vi "Sequence Execution.vi"() -> ()   [LabVIEW 2013, in "Simple Sequence Tools - Execution.lvlib"]
uses:
  Simple Sequence Tools - Execution.lvlib
  Types/Log.SelectedChannels.ctl
  Types/Execute.PreviewMode.ctl
  Types/Main.StateVariables.ctl
  Types/Execute.UserEventRefs.ctl
  <vilib>/NI Veristand/Execution/Workspace/SystemStateRegEventRef.ctl
  Types/Execution.SequenceState.ctl
  <vilib>/NI Veristand/Execution/DataLogging/DataLoggingSpecification Ref.ctl
  <vilib>/NI Veristand/Execution/DataLogging/IDataLogging Ref.ctl
  <vilib>/NI Veristand/Execution/Workspace/WorkspaceAPI.ctl
  <vilib>/NI Veristand/Execution/Workspace/SystemStateEventRef.ctl
  Shared/Types/INI.Settings
  NationalInstruments.VeriStand.RealTimeSequenceDefinitionApi
  Types/Results.Value.ctl
  Shared/SubVIs/Main.Constants.vi
  <vilib>/NI Veristand/Execution/Workspace/NI VeriStand - Set Single Channel Value.vi
  <vilib>/NI Veristand/Execution/Workspace/NI_VS Workspace ExecutionAPI.lvlib
  NationalInstruments.VeriStand.ClientAPI
  Shared/Simple Sequence Tools - Shared.lvlib
  <vilib>/NI Veristand/Execution/DataLogging/NI_VS Data Logging API.lvlib
panel:
  out "Duration":dbl min=1.0 max=3.0
  in  "Skip":bool
  out "Total Iterations":u32 min=1 max=2
  out "Current Step":u32 min=1 max=5
  out "Current Iteration":u32 min=1 max=2
  in  "NIVS.Gateway IP Address":string="localhost"
  in  "NIVS.Workspace Event":refnum<event-registration>
  in  "Preview Mode":T1=enum."Table"
  in  "Start Step":u32 min=1 max=11
  in  "Start Iteration":u32 min=1 max=5
  in  "Log Channels":T2=enum."Aliases"
  in  "Base File Name":string="Log" caption="Base File Name (timestamp included automatically)"
  in  "Enable Logging":bool=TRUE
  in  "Abort":bool
  in  "Pause":bool
  in  "Run":bool
  in  "Profiles":string(combo)
  out "Graph":waveform(dbl)[](graph)
  out "Sequence":i32[](listbox)=[-1]
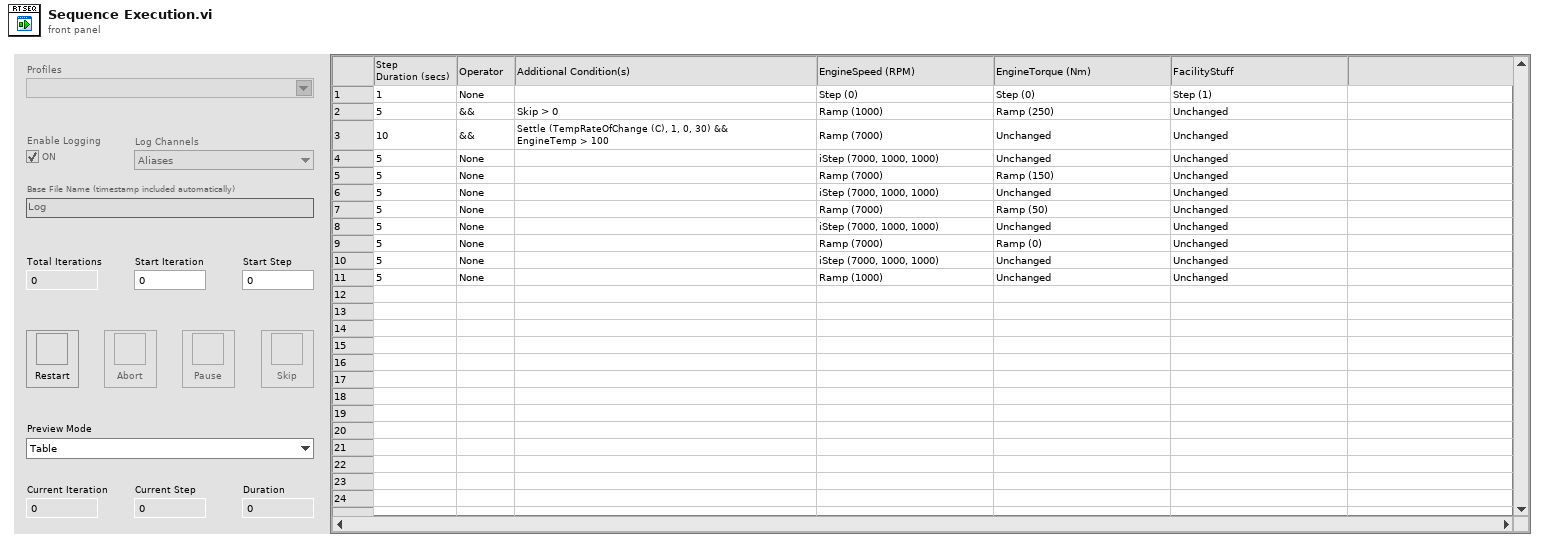
[diagram p1: front panel]
types:
  T1 = typedef "Simple Sequence Tools - Execution.lvlib/Execute.PreviewMode.ctl" = enum8{"Graph", "Table"}
  T2 = typedef "Simple Sequence Tools - Execution.lvlib/Log.SelectedChannels.ctl" = enum16{"Channels (No System Channel)", "Aliases", "All"}
  T3 = typedef "Simple Sequence Tools - Execution.lvlib/Execution.SequenceState.ctl" = enum16{"Idle", "Initializing", "Running", "Paused", "Finalizing", "Complete"}
  T4 = typedef "Simple Sequence Tools - Execution.lvlib/Main.StateVariables.ctl" = cluster{"NIVS.BaseLogPath":path, "NIVS.SystemDefinitionFile":path, "NIVS.Events":T5, "NIVS.SequenceState":T3, "NIVS.GatewayIPAddress":string, "NIVS.DataLogSpecRef":T7, "NIVS.DataLogManagerRef":T8, "NIVS.LogSessionGUID":string, "NIVS.WorkspaceManager":T9, "NIVS.Deployed":bool, "NIVS.ProfileRef":refnum<k24>, "NIVS.ProfileCallback":refnum<k27>, "NIVS.SystemStateRefs":T10, "UI.Abort":refnum<vi>, "UI.Pause":refnum<vi>, "UI.EnableLogging":refnum<vi>, "UI.Start":refnum<vi>, "UI.LogChannels":refnum<vi>, "UI.StartIteration":refnum<vi>, "UI.StartStep":refnum<vi>, "UI.Sequence":refnum<vi>, "UI.PreviewMode":refnum<vi>, "UI.Graph":refnum<vi>, "UI.BaseFileName":refnum<vi>, "UI.Profiles":refnum<vi>, "UI.CurrentStep":refnum<vi>, "UI.CurrentIteration":refnum<vi>, "UI.TotalIterations":refnum<vi>, "Sequence.AbortChannel":string, "Sequence.StepInfoChannel":string, "Sequence.Iterations":u32, "Sequence.IterationInfoChannel":string, "Sequence.#ofColumns":i32, "Events.State":refnum<user-event>, "Events.Test Result":refnum<user-event>, "Events.Progress":refnum<user-event>, "INI.Settings":T11, "UI.Skip":refnum<vi>, "Sequence.SkipChannel":string, "Restart.Path":path, "UI.Duration":refnum<vi>, "Sequence.DurationChannel":string}
  T5 = typedef "Simple Sequence Tools - Execution.lvlib/Execute.UserEventRefs.ctl" = cluster{"SequenceEvent":refnum<event-registration>, "SystemChangeEvent":T6, "WorkspaceEvent":refnum<event-registration>}
  T6 = typedef "NI_VS Workspace ExecutionAPI.lvlib/SystemStateRegEventRef.ctl" = refnum<event-registration>
  T7 = typedef "NI_VS Data Logging API.lvlib/DataLoggingSpecification Ref.ctl" = refnum<k24>
  T8 = typedef "NI_VS Data Logging API.lvlib/IDataLogging Ref.ctl" = refnum<k24>
  T9 = typedef "NI_VS Workspace ExecutionAPI.lvlib/WorkspaceAPI.ctl" = refnum<k24>
  T10 = typedef "NI_VS Workspace ExecutionAPI.lvlib/SystemStateEventRef.ctl" = cluster{"CustDatRef":refnum<user-event>, "EvtRef":refnum<k27>}
  T11 = typedef "Simple Sequence Tools - Shared.lvlib/INI.Settings" = cluster{"Build Location":path, "LoggingLocation":path}
  T12 = typedef "Simple Sequence Tools - Execution.lvlib/Results.Value.ctl" = enum8{"Passed", "Failed", "Aborted"}
  T13 = enum8{"Enabled", "Disabled", "Disabled and Grayed Out"}
  T14 = typedef "NI_VS Workspace ExecutionAPI.lvlib/SystemState.ctl" = u8
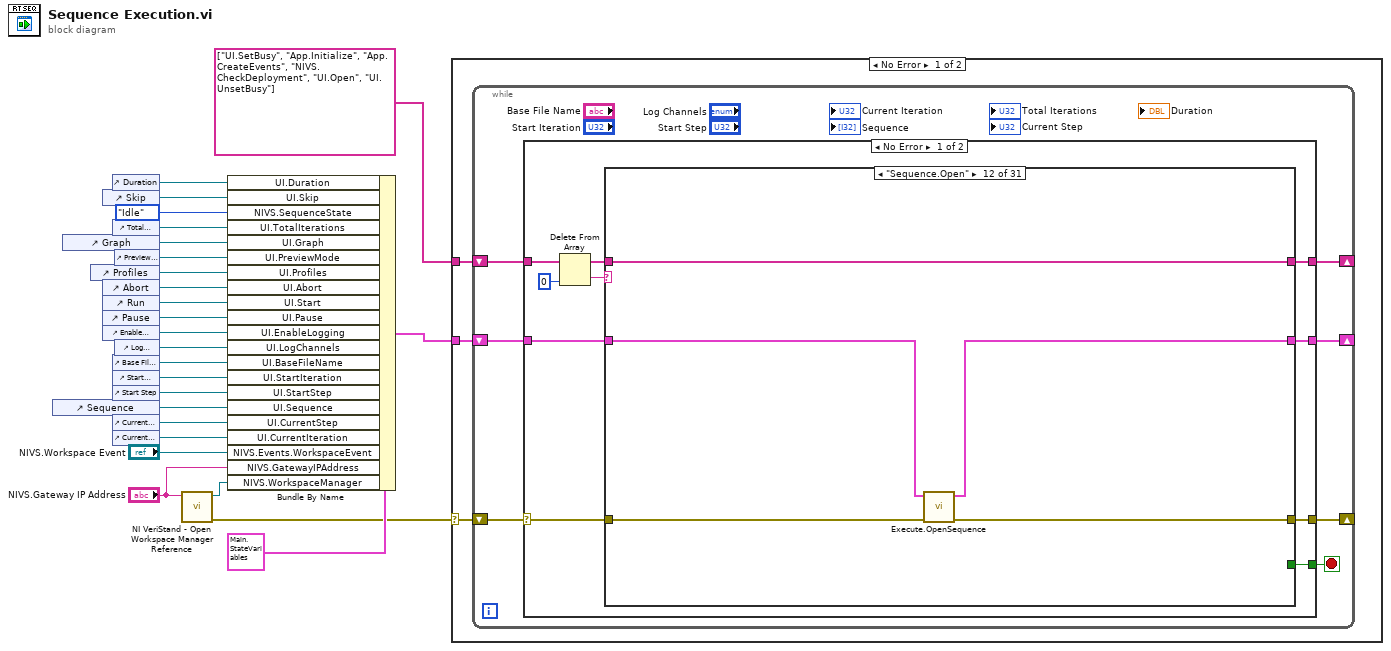
[diagram p0: block diagram]
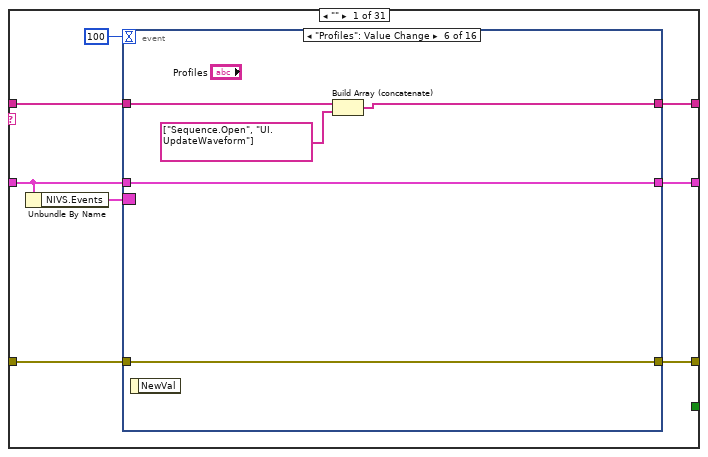
[diagram p2: hidden frame]
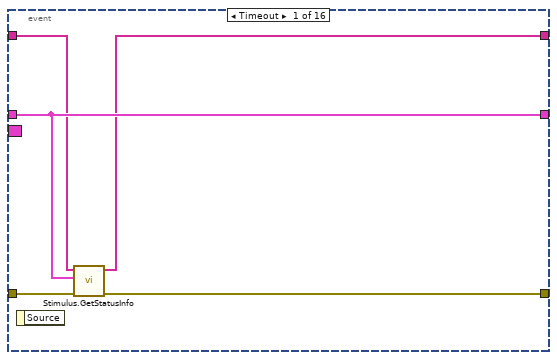
[diagram p3: hidden frame]
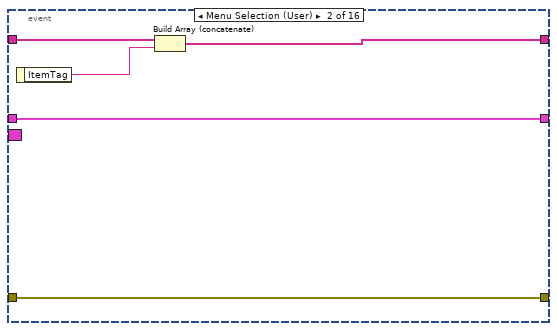
[diagram p4: hidden frame]
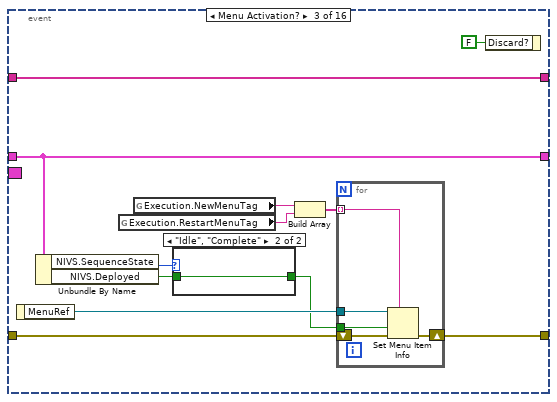
[diagram p5: hidden frame]
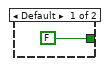
[diagram p6: hidden frame]
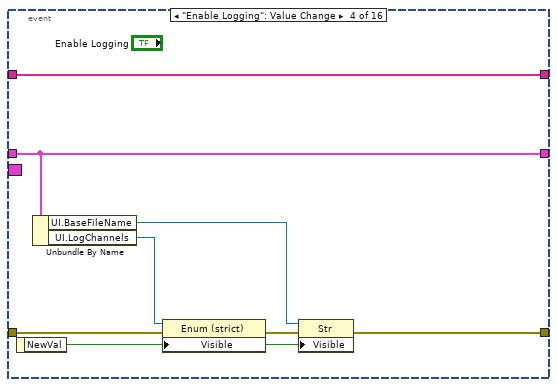
[diagram p7: hidden frame]
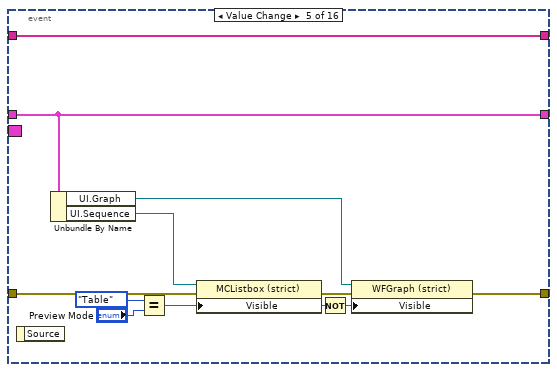
[diagram p8: hidden frame]
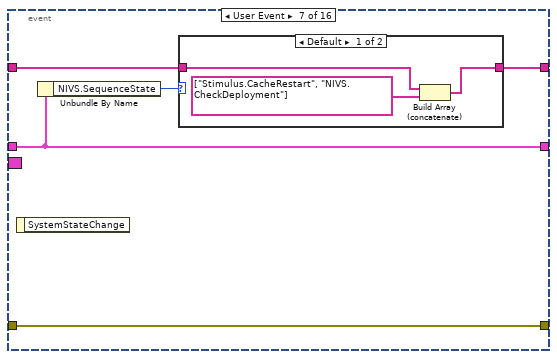
[diagram p9: hidden frame]
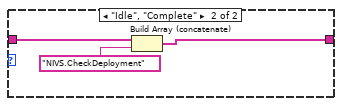
[diagram p10: hidden frame]
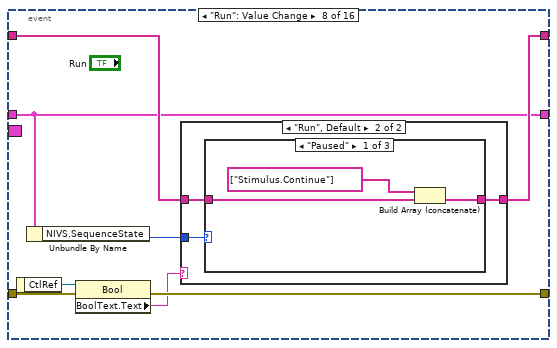
[diagram p11: hidden frame]
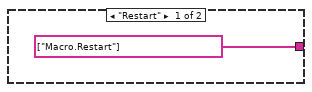
[diagram p12: hidden frame]
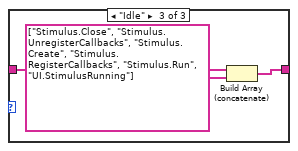
[diagram p14: hidden frame]
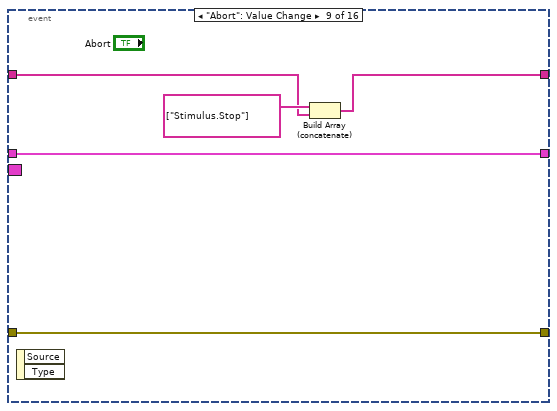
[diagram p15: hidden frame]
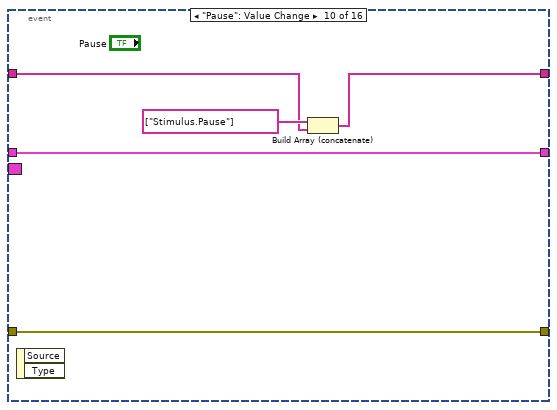
[diagram p16: hidden frame]
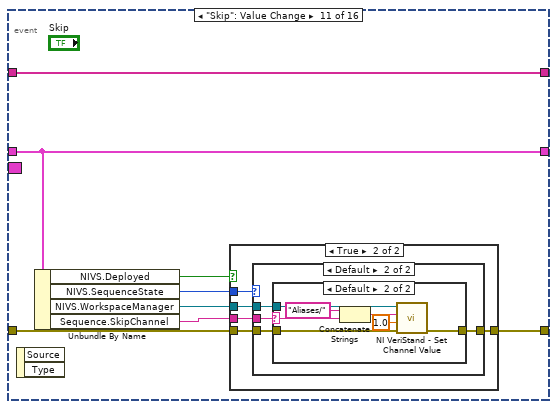
[diagram p17: hidden frame]
diagram:
  n1 = control-ref of="Sequence"() -> (w15:refnum<vi>)
  n2 = control-ref of="Graph"() -> (w24:refnum<vi>)
  n3 = control-ref of="Profiles"() -> (w13:refnum<vi>)
  n4 = control-ref of="Skip"() -> (w2:refnum<vi>)
  n5 = control-ref of="Abort"() -> (w22:refnum<vi>)
  n6 = control-ref of="Run"() -> (w21:refnum<vi>)
  n7 = control-ref of="Pause"() -> (w20:refnum<vi>)
  n8 = control-ref of="Enable Logging"() -> (w19:refnum<vi>)
  n9 = control-ref of="Duration"() -> (w1:refnum<vi>)
  n10 = control-ref of="Total Iterations"() -> (w6:refnum<vi>)
  n11 = control-ref of="Base File Name"() -> (w5:refnum<vi>)
  n12 = control-ref of="Start Iteration"() -> (w17:refnum<vi>)
  n13 = control-ref of="Start Step"() -> (w16:refnum<vi>)
  n14 = control-ref of="Current Step"() -> (w8:refnum<vi>)
  n15 = control-ref of="Current Iteration"() -> (w7:refnum<vi>)
  n16 = control-ref of="Preview Mode"() -> (w23:refnum<vi>)
  n17 = control-ref of="Log Channels"() -> (w18:refnum<vi>)
  n18 = call <vilib>:"NI VeriStand - Open Workspace Manager Reference.vi"("Gateway IP Address (\"\": localhost)"="NIVS.Gateway IP Address") -> ("error out"=w4:errorcluster, "WorkspaceManager"=w9:T9)  [unwired: 9 in]
  n19 = Bundle By Name(cluster=T4 {"NIVS.BaseLogPath"=path "", "NIVS.SystemDefinitionFile"=path "", "NIVS.Events"={"SequenceEvent"=refnum, "SystemChangeEvent"=refnum, "WorkspaceEvent"=refnum}, "NIVS.SequenceState"=enum."Idle", "NIVS.GatewayIPAddress"="", "NIVS.DataLogSpecRef"=refnum, "NIVS.DataLogManagerRef"=refnum, "NIVS.LogSessionGUID"="", "NIVS.WorkspaceManager"=refnum, "NIVS.Deployed"=FALSE, "NIVS.ProfileRef"=refnum, "NIVS.ProfileCallback"=refnum, "NIVS.SystemStateRefs"={"CustDatRef"=refnum, "EvtRef"=refnum}, "UI.Abort"=refnum, "UI.Pause"=refnum, "UI.EnableLogging"=refnum, "UI.Start"=refnum, "UI.LogChannels"=refnum, "UI.StartIteration"=refnum, "UI.StartStep"=refnum, "UI.Sequence"=refnum, "UI.PreviewMode"=refnum, "UI.Graph"=refnum, "UI.BaseFileName"=refnum, "UI.Profiles"=refnum, "UI.CurrentStep"=refnum, "UI.CurrentIteration"=refnum, "UI.TotalIterations"=refnum, "Sequence.AbortChannel"="", "Sequence.StepInfoChannel"="", "Sequence.Iterations"=0, "Sequence.IterationInfoChannel"="", "Sequence.#ofColumns"=0, "Events.State"=refnum, "Events.Test Result"=refnum, "Events.Progress"=refnum, "INI.Settings"={"Build Location"=path "", "LoggingLocation"=path ""}, "UI.Skip"=refnum, "Sequence.SkipChannel"="", "Restart.Path"=path "", "UI.Duration"=refnum, "Sequence.DurationChannel"=""} ("Cluster"), "UI.Duration"=w1, "UI.Skip"=w2, "NIVS.SequenceState"=Execution.SequenceState."Idle", "UI.TotalIterations"=w6, "UI.Graph"=w24, "UI.PreviewMode"=w23, "UI.Profiles"=w13, "UI.Abort"=w22, "UI.Start"=w21, "UI.Pause"=w20, "UI.EnableLogging"=w19, "UI.LogChannels"=w18, "UI.BaseFileName"=w5, "UI.StartIteration"=w17, "UI.StartStep"=w16, "UI.Sequence"=w15, "UI.CurrentStep"=w8, "UI.CurrentIteration"=w7, "NIVS.Events.WorkspaceEvent"="NIVS.Workspace Event", "NIVS.GatewayIPAddress"="NIVS.Gateway IP Address", "NIVS.WorkspaceManager"=w9) -> (w14:T4)
  n20 = case shown="No Error" w4 {
    selector: w4 -> [w26 _]
    tunnel: string[] ["UI.SetBusy", "App.Initialize", "App.CreateEvents", "NIVS.CheckDeployment", "UI.Open", "UI.UnsetBusy"] -> [w28 _]
    tunnel: w14 -> [w27 _]
    frame No Error {
      n21 = while {
        shift-right: [w34] -> _
        shift-left: w28 -> [w35]
        shift-right: [w32] -> _
        shift-left: w27 -> [w33]
        shift-right: [w30] -> _
        shift-left: w26 -> [w31]
        stop <- w29 stop-if-true
        n22 = case shown="No Error" w31 {
          selector: w31 -> [w36 w531]
          tunnel: w35 -> [w38 w534]
          tunnel: [w44 w534] -> w34
          tunnel: w33 -> [w42 w533]
          tunnel: [w41 w533] -> w32
          tunnel: [w40 w530] -> w30
          tunnel: [w39 _] -> w29
          frame No Error {
            n23 = Delete From Array(array=w38, index=0) -> (deleted portion=w45:string, array with subset deleted=w43:string[])  [unwired: 1 in]
            n24 = case shown="\"Sequence.Open\"" w45 {
              tunnel: [w51 w229 w242 w246 w258 w277 w286 w292 w295 w300 w322 w356 w361 w374 w379 w384 w390 w400 w412 w435 w450 w454 w458 w461 w464 w468 w472 w476 w491 w507 w529] -> w44
              tunnel: w43 -> [w50 w229 w242 w246 w259 w277 w286 w293 w296 w301 w323 w356 w361 w374 w379 w384 w390 w400 w412 w435 w450 w454 w458 w461 w464 w468 w472 w476 w491 w507 w529]
              tunnel: w42 -> [w47 w228 w238 w243 w251 w281 w287 w291 w298 w302 w325 w353 w358 w365 w376 w381 w389 w399 w409 w437 w446 w452 w457 w460 w463 w465 w469 w473 w490 w501 w528]
              tunnel: [w53 w232 w240 w243 w260 w281 w287 w291 w298 w302 w324 w352 w357 w366 w375 w380 w389 w399 w409 w437 w444 w452 w457 w460 w463 w465 w469 w473 w490 w501 w528] -> w41
              tunnel: [w48 w233 w241 w244 w255 w285 w289 w294 w299 w304 w320 w354 w359 w372 w378 w382 w385 w395 w410 w434 w448 w453 w455 w459 w462 w466 w470 w474 w481 w505 w527] -> w40
              tunnel: w36 -> [w49 w234 w239 w245 w256 w285 w289 w294 w299 w304 w321 w355 w360 w373 w377 w383 w386 w396 w411 w434 w449 w453 w456 w459 w462 w467 w471 w475 w480 w506 w527]
              tunnel: [_ _ _ _ _ _ TRUE _ _ _ _ _ _ _ _ _ _ _ _ _ _ _ _ _ _ _ _ _ _ _ _] -> w39
              frame "" {
                n25 = Unbundle By Name(w47) -> ("NIVS.Events"=w46:T5)
                n26 = event shown="[5] \"Profiles\": Value Change" {
                  selector: w46 -> [_ _ _ _ _ _ _ _ _ _ _ _ _ _ _ _]
                  dyn-events: _ -> [_ _ _ _ _ _ _ _ _ _ _ _ _ _ _ _]
                  timeout: 100 -> [_ _ _ _ _ _ _ _ _ _ _ _ _ _ _ _]
                  tunnel: [w55 w60 w75 w90 w101 w105 w110 w124 w137 w142 w154 w176 w191 w193 w203 w220] -> w51
                  tunnel: w50 -> [w56 w63 w75 w90 w101 w106 w111 w125 w138 w143 w154 w176 w192 w194 w206 w223]
                  tunnel: [w58 w62 w74 w89 w98 w104 w108 w123 w141 w146 w153 w175 w182 w196 w201 w219] -> w53
                  tunnel: w47 -> [w58 w62 w74 w89 w98 w104 w108 w123 w141 w146 w153 w175 w183 w197 w201 w219]
                  tunnel: [w54 w61 w70 w83 w91 w103 w109 w119 w140 w145 w149 w174 w184 w199 w207 w222] -> w48
                  tunnel: w49 -> [w57 w61 w71 w87 w92 w103 w109 w120 w140 w145 w150 w174 w187 w199 w207 w222]
                  event Timeout {
                    n27 = event-data() -> ()  [unwired: 1 in, 1 out]
                    n28 = call "Stimulus.GetStatusInfo.vi"("error in (no error)"=w57, "Cluster"=w58, "Commands"=w56) -> ("error out"=w54:errorcluster, "Commands out"=w55:string[])  [unwired: 7 in]
                  }
                  event Menu Selection (User) {
                    n29 = event-data() -> ("ItemTag"=w59:string)  [unwired: 1 in]
                    n30 = Build Array (concatenate)(w63, w59) -> (w60:string[])
                  }
                  event Menu Activation? {
                    n31 = event-data() -> ("MenuRef"=w72:refnum<k9>)  [unwired: 1 in]
                    n32 = Unbundle By Name(w74) -> ("NIVS.SequenceState"=w73:T3, "NIVS.Deployed"=w64:bool)
                    n33 = global read "Main.Constants.vi" "Execution.RestartMenuTag"() -> (w67:string)
                    n34 = global read "Main.Constants.vi" "Execution.NewMenuTag"() -> (w68:string)
                    n35 = case shown="\"Idle\", \"Complete\"" w73 {
                      tunnel: [FALSE w82] -> w69
                      tunnel: w64 -> [_ w82]
                      frame Default {
                      }
                      frame "Idle", "Complete" {
                      }
                    }
                    n36 = Build Array(w68, w67) -> (w66:string[])
                    n37 = for {
                      tunnel: w72 -> [w80]
                      shift-right: [w78] -> w70
                      shift-left: w71 -> [w79]
                      tunnel: w69 -> [w77]
                      tunnel: w66 -> [w76] mode=indexing
                      n38 = Set Menu Item Info(7:w76, 8:w79, 9:w77, 11:w80) -> (0:w78:errorcluster)  [unwired: 3 in, 1 out]
                    }
                    n39 = event-data("Discard?"=FALSE) -> ()  [unwired: 1 in, 1 out]
                  }
                  event "Enable Logging": Value Change {
                    n40 = event-data() -> ("NewVal"=w84:bool)  [unwired: 1 in]
                    n41 = Unbundle By Name(w89) -> ("UI.BaseFileName"=w85:refnum<vi>, "UI.LogChannels"=w88:refnum<vi>)
                    n42 = property class="Enum (strict)"(reference=w88, error in=w87, "Visible"=w84) -> (error out=w86:errorcluster)  [unwired: 1 out]
                    n43 = property class="Str"(reference=w85, error in=w86, "Visible"=w84) -> (error out=w83:errorcluster)  [unwired: 1 out]
                  }
                  event Value Change {
                    n44 = event-data() -> ()  [unwired: 1 in, 1 out]
                    n45 = Unbundle By Name(w98) -> ("UI.Graph"=w96:refnum<vi>, "UI.Sequence"=w97:refnum<vi>)
                    n46 = Equal?(x=Execute.PreviewMode."Table" ("y"), y="Preview Mode") -> (x = y?=w94:bool)
                    n47 = property class="MCListbox (strict)"(reference=w97, error in=w92, "Visible"=w94) -> (error out=w95:errorcluster)  [unwired: 1 out]
                    n48 = Not(x=w94) -> (.not. x?=w93:bool)
                    n49 = property class="WFGraph (strict)"(reference=w96, error in=w95, "Visible"=w93) -> (error out=w91:errorcluster)  [unwired: 1 out]
                  }
                  event "Profiles": Value Change {
                    n50 = event-data() -> ()  [unwired: 1 in, 1 out]
                    n51 = Build Array (concatenate)(w106, string[] ["Sequence.Open", "UI.UpdateWaveform"]) -> (w105:string[])
                  }
                  event User Event {
                    n52 = event-data() -> ()  [unwired: 1 in, 1 out]
                    n53 = Unbundle By Name(w108) -> ("NIVS.SequenceState"=w107:T3)
                    n54 = case shown="Default" w107 {
                      tunnel: w111 -> [w113 w117]
                      tunnel: [w112 w116] -> w110
                      frame Default {
                        n55 = Build Array (concatenate)(w113, string[] ["Stimulus.CacheRestart", "NIVS.CheckDeployment"]) -> (w112:string[])
                      }
                      frame "Idle", "Complete" {
                        n56 = Build Array (concatenate)(w117, "NIVS.CheckDeployment") -> (w116:string[])
                      }
                    }
                  }
                  event "Run": Value Change {
                    n57 = event-data() -> ("CtlRef"=w121:refnum<vi>)  [unwired: 1 in]
                    n58 = Unbundle By Name(w123) -> ("NIVS.SequenceState"=w122:T3)
                    n59 = property class="Bool"(reference=w121, error in=w120) -> (error out=w119:errorcluster, "BoolText.Text"=w118:string)  [unwired: 1 out]
                    n60 = case shown="\"Run\", Default" w118 {
                      tunnel: w125 -> [_ w129]
                      tunnel: [string[] ["Macro.Restart"] w128] -> w124
                      tunnel: w122 -> [_ w127]
                      frame "Restart" {
                      }
                      frame "Run", Default {
                        n61 = case shown="\"Paused\"" w127 {
                          tunnel: w129 -> [w131 w133 w136]
                          tunnel: [w130 w133 w135] -> w128
                          frame "Paused" {
                            n62 = Build Array (concatenate)(string[] ["Stimulus.Continue"] ("array"), w131) -> (w130:string[])
                          }
                          frame Default {
                          }
                          frame "Idle" {
                            n63 = Build Array (concatenate)(w136, string[] ["Stimulus.Close", "Stimulus.UnregisterCallbacks", "Stimulus.Create", "Stimulus.RegisterCallbacks", "Stimulus.Run", "UI.StimulusRunning"] ("array")) -> (w135:string[])
                          }
                        }
                      }
                    }
                  }
                  event "Abort": Value Change {
                    n64 = event-data() -> ()  [unwired: 1 in, 2 out]
                    n65 = Build Array (concatenate)(string[] ["Stimulus.Stop"] ("array"), w138) -> (w137:string[])
                  }
                  event "Pause": Value Change {
                    n66 = event-data() -> ()  [unwired: 1 in, 2 out]
                    n67 = Build Array (concatenate)(string[] ["Stimulus.Pause"] ("array"), w143) -> (w142:string[])
                  }
                  event "Skip": Value Change {
                    n68 = event-data() -> ()  [unwired: 1 in, 2 out]
                    n69 = Unbundle By Name(w153) -> ("NIVS.Deployed"=w148:bool, "NIVS.SequenceState"=w147:T3, "NIVS.WorkspaceManager"=w152:T9, "Sequence.SkipChannel"=w151:string)
                    n70 = case shown="True" w148 {
                      tunnel: w152 -> [_ w158]
                      tunnel: w150 -> [w155 w160]
                      tunnel: [w155 w159] -> w149
                      tunnel: w151 -> [_ w157]
                      tunnel: w147 -> [_ w156]
                      frame False {
                      }
                      frame True {
                        n71 = case shown="Default" w156 {
                          tunnel: w160 -> [w161 w165]
                          tunnel: [w161 w164] -> w159
                          tunnel: w158 -> [_ w163]
                          tunnel: w157 -> [_ w162]
                          frame "Idle", "Complete" {
                          }
                          frame Default {
                            n72 = case shown="Default" w162 {
                              selector: w162 -> [_ w168]
                              tunnel: w165 -> [w166 w173]
                              tunnel: [w166 w172] -> w164
                              tunnel: w163 -> [_ w171]
                              frame "" {
                              }
                              frame Default {
                                n73 = Concatenate Strings("Aliases/" ("string"), w168) -> (w167:string)
                                n74 = call-poly <vilib>:"NI VeriStand - Set Channel Value.vi"("error in (no error)"=w173, "Value"=1.0, "Channel"=w167, "WorkspaceManager in"=w171) -> ("error out"=w172:errorcluster)  [unwired: 6 in, 1 out]
                              }
                            }
                          }
                        }
                      }
                    }
                  }
                  event User Event {
                    n75 = event-data() -> ()  [unwired: 1 in, 2 out]
                  }
                  event User Event {
                    n76 = event-data() -> ("Test Result"=w186:path)  [unwired: 1 in]
                    n77 = Path To String(path=w186) -> (string=w189:string)
                    n78 = Concatenate Strings("explorer " ("string"), w189) -> (w177:string)
                    n79 = call <vilib>:"System Exec.vi"("error in (no error)"=w187, "command line"=w177) -> ("error out"=w185:errorcluster)  [unwired: 6 in, 3 out]
                    n80 = call "Restart.HandleSequenceFinishedEvent.vi"("error in (no error)"=w185, "results path"=w186, "State Variables"=w183) -> ("error out"=w184:errorcluster, "Restart?"=w181:bool, "State Variables out"=w182:T4)  [unwired: 6 in]
                    n81 = Select(t="UI.StimulusRestart", s=w181, f="UI.StimulusComplete") -> (s? t:f=w178:string)
                    n82 = Build Array (concatenate)(w192, string[] ["Stimulus.Close", "Stimulus.UnregisterCallbacks"], w178) -> (w191:string[])
                  }
                  event User Event {
                    n83 = event-data() -> ("State"=w198:i32)  [unwired: 1 in]
                    n84 = Bundle By Name(cluster=w197, "NIVS.SequenceState"=w198) -> (w196:T4)
                    n85 = Build Array (concatenate)(w194, string[] ["UI.UpdateState"] ("array")) -> (w193:string[])
                  }
                  event User Event {
                    n86 = event-data() -> ("Workspace Event"=w202:string)  [unwired: 1 in]
                    n87 = Unbundle By Name(w201) -> ("NIVS.SequenceState"=w200:T3)
                    n88 = Equal?(x="Shut Down" ("y"), y=w202) -> (x = y?=w204:bool)
                    n89 = case shown="False" w204 {
                      tunnel: w206 -> [w208 w211]
                      tunnel: [w208 w210] -> w203
                      tunnel: w200 -> [_ w209]
                      frame False {
                      }
                      frame True {
                        n90 = case shown="Default" w209 {
                          tunnel: w211 -> [w213 w217]
                          tunnel: [w212 w215] -> w210
                          frame Default {
                            n91 = Build Array (concatenate)(w213, string[] ["Stimulus.CacheRestart", "Macro.Exit"]) -> (w212:string[])
                          }
                          frame "Idle", "Complete" {
                            n92 = Build Array (concatenate)(w217, "Macro.Exit" ("y")) -> (w215:string[])
                          }
                        }
                      }
                    }
                  }
                  event Panel Close? {
                    n93 = event-data() -> ()  [unwired: 1 in, 1 out]
                    n94 = Build Array (concatenate)(w223, "Macro.Exit") -> (w220:string[])
                    n95 = event-data("Discard?"=TRUE) -> ()  [unwired: 1 in, 1 out]
                  }
                }
              }
              frame "App.Initialize" {
                n96 = Unbundle By Name(w228) -> ("NIVS.Events.WorkspaceEvent"=w227:refnum<event-registration>)
                n97 = call "Execute.Initialize.vi"("error in (no error)"=w234, "Cluster"=w228) -> ("error out"=w230:errorcluster)  [unwired: 9 in]
                n98 = Not A Number/Path/Refnum?(number/path/refnum=w227) -> (NaN/Path/Refnum?=w225:bool)
                n99 = case shown="False" w225 {
                  tunnel: [w235 w237] -> w226
                  frame False {
                    n100 = property class="VI"() -> ("Path"=w236:path)  [unwired: 2 in, 2 out]
                    n101 = Strip Path(path=w236) -> (stripped path=w235:path)  [unwired: 1 out]
                  }
                  frame True {
                    n102 = call <vilib>:"Application Directory.vi"() -> ("Application Directory"=w237:path)
                  }
                }
                n103 = call "INI.GetSettings.vi"("error in (no error)"=w230, "INI Folder Location"=w226) -> ("error out"=w233:errorcluster, "INI.Settings"=w231:T11)  [unwired: 8 in]
                n104 = Bundle By Name(cluster=w228, "Restart.Path"=path "", "INI.Settings"=w231) -> (w232:T4)
              }
              frame "App.CreateEvents" {
                n105 = call "Execute.CreateEvents.vi"("error in (no error)"=w239, "Cluster in"=w238) -> ("error out"=w241:errorcluster, "Cluster out"=w240:T4)  [unwired: 8 in]
              }
              frame "App.LoadSequences" {
                n106 = call "Execute.LoadSequences.vi"("error in (no error)"=w245, "Cluster"=w243) -> ("error out"=w244:errorcluster)  [unwired: 9 in]
              }
              frame "App.Restart" {
                n107 = Unbundle By Name(w251) -> ("NIVS.BaseLogPath"=w250:path)
                n108 = call "File Dialog"("start path"=w250, "prompt"="Select the restart file.", "button label"="Select", "error in"=w256, "pattern (all files)"="*.info", "pattern label"="Restart Info") -> ("selected path"=w253:path, "cancelled"=w257:bool, "error out"=w254:errorcluster)  [unwired: 6 in, 1 out]
                n109 = case shown="False" w257 {
                  tunnel: w251 -> [w263 w275]
                  tunnel: [w268 w275] -> w260
                  tunnel: w259 -> [w267 w276]
                  tunnel: [w266 w276] -> w258
                  tunnel: [w265 w273] -> w255
                  tunnel: w254 -> [w264 w274]
                  tunnel: w253 -> [w262 _]
                  frame False {
                    n110 = call "Restart.CheckValidSelection.vi"("error in (no error)"=w264, "Restart Path"=w262, "State Variables"=w263) -> ("error out"=w265:errorcluster, "Load Restart?"=w261:bool, "State Variables out"=w268:T4)  [unwired: 6 in]
                    n111 = case shown="True" w261 {
                      tunnel: w267 -> [w269 w272]
                      tunnel: [w269 w271] -> w266
                      frame False {
                      }
                      frame True {
                        n112 = Build Array (concatenate)(w272, "UI.StimulusRestart") -> (w271:string[])
                      }
                    }
                  }
                  frame True {
                    n113 = call <vilib>:"Clear Errors.vi"("error in (no error)"=w274) -> ("error out"=w273:errorcluster)  [unwired: 6 in]
                  }
                }
              }
              frame "App.CloseReferences" {
                n114 = Unbundle By Name(w281) -> ("Events.State"=w282:refnum<user-event>, "Events.Test Result"=w283:refnum<user-event>, "Events.Progress"=w284:refnum<user-event>, "NIVS.Events"=w280:T5, "NIVS.SystemStateRefs"=w279:T10, "NIVS.WorkspaceManager"=w278:T9)
                n115 = disable-structure shown="Enabled" {
                  frame Enabled {
                    n116 = invoke class="VI" method="FP.Close"() -> ()  [unwired: 3 in, 3 out]
                  }
                  frame Disabled {
                  }
                }
                n117 = call <vilib>:"NI VeriStand - Close Workspace Manager Reference.vi"("WorkspaceManager"=w278) -> ()  [unwired: 10 in, 1 out]
                n118 = call <vilib>:"NI VeriStand - Close Engine State Change Notification.vi"("SystemStateRefs"=w279) -> ()  [unwired: 10 in, 1 out]
                n119 = Unregister For Events(event registration refnum=w280) -> ()  [unwired: 1 in, 1 out]
                n120 = Destroy User Event(user event=w284) -> ()  [unwired: 1 in, 1 out]
                n121 = Destroy User Event(user event=w283) -> ()  [unwired: 1 in, 1 out]
                n122 = Destroy User Event(user event=w282) -> ()  [unwired: 1 in, 1 out]
              }
              frame "App.Exit" {
              }
              frame "Macro.New" {
                n123 = Build Array (concatenate)(w293, string[] ["UI.SetBusy", "App.Initialize", "NIVS.CheckDeployment", "UI.UnsetBusy"]) -> (w292:string[])
              }
              frame "Macro.Restart" {
                n124 = Build Array (concatenate)(w296, string[] ["Stimulus.Close", "Stimulus.UnregisterCallbacks", "Stimulus.Open", "Stimulus.RegisterCallbacks", "Stimulus.Run", "UI.StimulusRunning"] ("array")) -> (w295:string[])
              }
              frame "Macro.Exit" {
                n125 = Unbundle By Name(w302) -> ("NIVS.SequenceState"=w303:T3)
                n126 = case shown="\"Idle\", \"Complete\"" w303 {
                  tunnel: w301 -> [w307 w310]
                  tunnel: [w305 w309] -> w300
                  frame "Idle", "Complete" {
                    n127 = Build Array (concatenate)(w307, string[] ["Stimulus.Stop", "Stimulus.Close", "Stimulus.UnregisterCallbacks", "App.CloseReferences", "App.Exit"]) -> (w305:string[])
                  }
                  frame Default {
                    n128 = Two Button Dialog(message="A test is running and exiting will abort the test. Do you want to exit?", 1:"No" ("F button name (\"Cancel\")"), 2:"Yes" ("T button name (\"OK\")")) -> (T button?=w308:bool)
                    n129 = case shown="True" w308 {
                      tunnel: w310 -> [w314 w317]
                      tunnel: [w314 w315] -> w309
                      frame False {
                      }
                      frame True {
                        n130 = Build Array (concatenate)(w317, string[] ["Stimulus.Stop", "Stimulus.Close", "Stimulus.CacheRestart", "Stimulus.UnregisterCallbacks", "App.CloseReferences", "App.Exit"]) -> (w315:string[])
                      }
                    }
                  }
                }
              }
              frame "NIVS.CheckDeployment" {
                n131 = Unbundle By Name(w325) -> ("INI.Settings.LoggingLocation"=w319:path, "NIVS.WorkspaceManager"=w326:T9)
                n132 = call <vilib>:"NI VeriStand - Get System State.vi"("error in (no error)"=w321, "WorkspaceManager in"=w326) -> ("error out"=w320:errorcluster, "System State"=w327:T14, "System Definition File"=w318:path)  [unwired: 5 in, 2 out]
                n133 = case shown="1" w327 {
                  tunnel: w323 -> [w331 w345]
                  tunnel: [w330 w344] -> w322
                  tunnel: w325 -> [w334 w342]
                  tunnel: [w333 w340] -> w324
                  tunnel: w319 -> [_ w337]
                  tunnel: w318 -> [_ w336]
                  frame 0, Default {
                    w328 = path ""
                    # "Not connected"
                    n134 = Bundle By Name(cluster=w334, "NIVS.Deployed"=FALSE ("Connected"), "NIVS.SystemDefinitionFile"=w328, "NIVS.BaseLogPath"=w328) -> (w333:T4)
                    n135 = Build Array (concatenate)(w331, "App.Initialize") -> (w330:string[])
                  }
                  frame 1 {
                    # "Connected"
                    n136 = Empty String/Path?(string/path=w337) -> (empty?=w338:bool)
                    n137 = case shown="True" w338 {
                      tunnel: [w347 w349] -> w339
                      tunnel: w337 -> [w347 _]
                      tunnel: w336 -> [w346 w348]
                      tunnel: [w346 w348] -> w335
                      frame False {
                      }
                      frame True {
                        n138 = Strip Path(path=w348) -> (stripped path=w351:path)  [unwired: 1 out]
                        n139 = Build Path(base path=w351, name or relative path="Logs") -> (appended path=w349:path)
                      }
                    }
                    n140 = Build Array (concatenate)(string[] ["App.LoadSequences", "UI.Connected"], w345) -> (w344:string[])
                    n141 = Bundle By Name(cluster=w342, "NIVS.Deployed"=TRUE ("Connected"), "NIVS.BaseLogPath"=w339, "NIVS.SystemDefinitionFile"=w335) -> (w340:T4)
                  }
                }
              }
              frame "Sequence.Open" {
                n142 = call "Execute.OpenSequence.vi"("error in (no error)"=w355, "State Variables"=w353) -> ("error out"=w354:errorcluster, "State Variables"=w352:T4)  [unwired: 8 in]
              }
              frame "Stimulus.Create" {
                n143 = call "Stimulus.Create.vi"("error in (no error)"=w360, "State Variables"=w358) -> ("error out"=w359:errorcluster, "State Variables"=w357:T4)  [unwired: 8 in]
              }
              frame "Stimulus.RegisterCallbacks" {
                n144 = Unbundle By Name(w365) -> ("NIVS.ProfileRef"=w371:refnum<k24>, "Events.Progress"=w370:refnum<user-event>, "Events.Test Result"=w369:refnum<user-event>, "Events.State"=w368:refnum<user-event>)
                n145 = vi-ref "SequenceEvent.ProgressChanged.vi"() -> ("vi reference"=w364:refnum<vi>)
                n146 = vi-ref "SequenceEvent.ExecuteCompleted.vi"() -> ("vi reference"=w363:refnum<vi>)
                n147 = vi-ref "SequenceEvent.PropertyChanged.vi"() -> ("vi reference"=w362:refnum<vi>)
                n148 = node(w373, w371, w364, w370, w371, w363, w369, w371, w362, w368) -> (w367:refnum<k27>, w372:errorcluster)  [unwired: 1 in]
                n149 = Bundle By Name(cluster=w365, "NIVS.ProfileCallback"=w367) -> (w366:T4)
              }
              frame "Stimulus.Run" {
                n150 = call "Stimulus.Run.vi"("error in (no error)"=w377, "Cluster in"=w376) -> ("error out"=w378:errorcluster, "Cluster out"=w375:T4)  [unwired: 8 in]
              }
              frame "Stimulus.Open" {
                n151 = call "Stimulus.Open.vi"("error in (no error)"=w383, "State Variables"=w381) -> ("error out"=w382:errorcluster, "State Variables"=w380:T4)  [unwired: 8 in]
              }
              frame "Stimulus.Pause" {
                n152 = Unbundle By Name(w389) -> ("NIVS.SequenceState"=w387:T3, "NIVS.ProfileRef"=w388:refnum<k24>)
                n153 = case shown="\"Running\"" w387 {
                  tunnel: w388 -> [_ w394]
                  tunnel: w386 -> [w391 w393]
                  tunnel: [w391 w392] -> w385
                  frame "Idle", Default {
                  }
                  frame "Running" {
                    n154 = invoke class="StimulusProfile" method="Pause"(reference=w394, error in=w393) -> (error out=w392:errorcluster)  [unwired: 1 in, 2 out]
                  }
                }
              }
              frame "Stimulus.Continue" {
                n155 = Unbundle By Name(w399) -> ("NIVS.SequenceState"=w398:T3, "NIVS.ProfileRef"=w397:refnum<k24>)
                n156 = case shown="\"Paused\"" w398 {
                  tunnel: w397 -> [_ w404]
                  tunnel: w396 -> [w401 w403]
                  tunnel: [w401 w402] -> w395
                  frame "Idle", Default {
                  }
                  frame "Paused" {
                    n157 = invoke class="StimulusProfile" method="Continue"(reference=w404, error in=w403) -> (error out=w402:errorcluster)  [unwired: 1 in, 2 out]
                  }
                }
              }
              frame "Stimulus.Stop" {
                n158 = Unbundle By Name(w409) -> ("NIVS.WorkspaceManager"=w405:T9, "Sequence.AbortChannel"=w406:string, "NIVS.SequenceState"=w407:T3, "NIVS.ProfileRef"=w408:refnum<k24>)
                n159 = case shown="\"Running\", \"Paused\", Default" w407 {
                  tunnel: w408 -> [_ w415]
                  tunnel: w411 -> [w413 w419]
                  tunnel: [w413 w414] -> w410
                  tunnel: w406 -> [_ w418]
                  tunnel: w405 -> [_ w417]
                  frame "Idle" {
                  }
                  frame "Running", "Paused", Default {
                    n160 = case shown="Default" w418 {
                      selector: w418 -> [_ w422]
                      tunnel: w419 -> [w420 w429]
                      tunnel: [w420 w425] -> w416
                      tunnel: w417 -> [_ w428]
                      frame "" {
                      }
                      frame Default {
                        n161 = Concatenate Strings("Aliases/" ("string"), w422) -> (w421:string)
                        n162 = call-poly <vilib>:"NI VeriStand - Set Channel Value.vi"("error in (no error)"=w429, "Value"=1.0, "Channel"=w421, "WorkspaceManager in"=w428) -> ("error out"=w426:errorcluster)  [unwired: 6 in, 1 out]
                        n163 = flat-sequence {
                          tunnel: w426 -> [w431]
                          tunnel: [w431] -> w425
                          tunnel: 100 -> [w430]
                          frame #0 {
                            n164 = Wait (ms)(milliseconds to wait=w430) -> ()  [unwired: 1 out]
                          }
                        }
                      }
                    }
                    n165 = invoke class="StimulusProfile" method="Stop"(reference=w415, error in=w416) -> (error out=w414:errorcluster)  [unwired: 1 in, 2 out]
                  }
                }
              }
              frame "Stimulus.Close" {
                n166 = Unbundle By Name(w437) -> ("NIVS.ProfileRef"=w436:refnum<k24>, "NIVS.DataLogManagerRef"=w433:T8, "NIVS.LogSessionGUID"=w432:string)
                n167 = case shown="Default" w432 {
                  selector: w432 -> [_ w439]
                  tunnel: w433 -> [_ w442]
                  tunnel: [_ w438] -> _
                  frame "" {
                  }
                  frame Default {
                    n168 = call <vilib>:"Stop Data Logging Session.vi"("Session Name in"=w439, "Data Logging Manager Ref in"=w442) -> ("error out"=w440:errorcluster, "Data Logging Manager Ref out"=w441:T8)  [unwired: 7 in, 1 out]
                    n169 = call <vilib>:"Close Data Logging Manager Reference.vi"("error in (no error)"=w440, "Data Logging Manager Ref in"=w441) -> ("error out"=w438:errorcluster)  [unwired: 9 in]
                  }
                }
                n170 = Close Reference(reference=w436) -> ()  [unwired: 1 in, 1 out]
              }
              frame "Stimulus.CacheRestart" {
                n171 = call "Restart.CacheCurrentLocation.vi"("error in (no error)"=w449, "Result"=Results.Value."Aborted", "State Variables"=w446) -> ("error out"=w448:errorcluster, "State Variables out"=w445:T4)  [unwired: 6 in, 1 out]
                n172 = Bundle By Name(cluster=w445, "Restart.Path"=path "") -> (w444:T4)
              }
              frame "Stimulus.UnregisterCallbacks" {
                n173 = Unbundle By Name(w452) -> ("NIVS.ProfileCallback"=w451:refnum<k27>)
                n174 = Unregister For Events(event registration refnum=w451) -> ()  [unwired: 1 in, 1 out]
              }
              frame "UI.Open" {
                n175 = invoke class="VI" method="FP.Open"(error in=w456) -> (error out=w455:errorcluster)  [unwired: 4 in, 4 out]
              }
              frame "UI.SetBusy" {
                n176 = call <vilib>:"Set Busy.vi"() -> ()  [unwired: 10 in, 2 out]
              }
              frame "UI.UnsetBusy" {
                n177 = call <vilib>:"Unset Busy.vi"() -> ()  [unwired: 11 in, 1 out]
              }
              frame "UI.StimulusComplete" {
                n178 = call "UI.StimulusComplete.vi"("error in (no error)"=w467, "Cluster"=w465) -> ("error out"=w466:errorcluster)  [unwired: 9 in]
              }
              frame "UI.StimulusRestart" {
                n179 = call "UI.StimulusRestart.vi"("error in (no error)"=w471, "Cluster"=w469) -> ("error out"=w470:errorcluster)  [unwired: 9 in]
              }
              frame "UI.StimulusRunning" {
                n180 = call "Execute.UI.Running.vi"("error in (no error)"=w475, "Cluster"=w473) -> ("error out"=w474:errorcluster)  [unwired: 9 in]
              }
              frame "UI.UpdateState" {
                n181 = Unbundle By Name(w490) -> ("UI.Start"=w483:refnum<vi>, "UI.Abort"=w484:refnum<vi>, "UI.Pause"=w488:refnum<vi>, "UI.Skip"=w478:refnum<vi>, "NIVS.SequenceState"=w489:T3)
                n182 = case shown="\"Idle\"" w489 {
                  tunnel: [w492 w494 T13."Disabled and Grayed Out" ("Disabled") w497] -> w477
                  tunnel: [T13."Disabled and Grayed Out" ("Disabled") w494 w496 T13."Enabled" ("f")] -> w482
                  tunnel: [w492 w494 w496 w497] -> w485
                  frame "Running" {
                    w492 = T13."Enabled" ("Disabled")
                  }
                  frame Default {
                    w494 = T13."Disabled and Grayed Out" ("Disabled")
                  }
                  frame "Paused" {
                    w496 = T13."Enabled" ("Disabled")
                  }
                  frame "Idle" {
                    w497 = T13."Disabled and Grayed Out" ("Disabled")
                  }
                }
                n183 = property class="Bool"(reference=w478, error in=w480, "DisabledEnum"=w477) -> (error out=w479:errorcluster)  [unwired: 1 out]
                n184 = property class="Bool"(reference=w488, error in=w479, "DisabledEnum"=w477) -> (error out=w487:errorcluster)  [unwired: 1 out]
                n185 = property class="Bool"(reference=w484, error in=w487, "DisabledEnum"=w485) -> (error out=w486:errorcluster)  [unwired: 1 out]
                n186 = property class="Bool"(reference=w483, error in=w486, "DisabledEnum"=w482) -> (error out=w481:errorcluster)  [unwired: 1 out]
              }
              frame "UI.UpdateWaveform" {
                n187 = Unbundle By Name(w501) -> ("NIVS.SequenceState"=w500:T3, "UI.Graph"=w502:refnum<vi>, "UI.Sequence"=w503:refnum<vi>, "Sequence.#ofColumns"=w504:i32)
                n188 = case shown="Default" w500 {
                  tunnel: w506 -> [w514 w521]
                  tunnel: [w513 w526] -> w505
                  tunnel: w504 -> [w511 w524]
                  tunnel: w503 -> [w510 w516]
                  tunnel: w502 -> [w509 w523]
                  tunnel: [w508 w522] -> w499
                  frame "Idle" {
                    n189 = call "Sequence.BuildPreviewWaveform.vi"("WaveformGraph in"=w509, "error in (no error)"=w514, "Rows"=cluster{"Start Index":i32, "Length":i32} {"Start Index"=0, "Length"=-1}, "UI.Sequence#ofColumns"=w511, "SequenceRef"=w510) -> ("error out"=w513:errorcluster, "Wavefrom"=w508:waveform(dbl)[])  [unwired: 5 in]
                  }
                  frame Default {
                    n190 = property class="MCListbox (strict)"(reference=w516, error in=w521) -> (reference out=w515:refnum<vi>, error out=w520:errorcluster, "Value"=w518:i32[])
                    n191 = Index Array(array=w518) -> (element=w517:i32)  [unwired: 1 in]
                    n192 = Bundle By Name(cluster=cluster{"Start Index":i32, "Length":i32} {"Start Index"=0, "Length"=1} ("Rows"), "Start Index"=w517) -> (w519:cluster{"Start Index":i32, "Length":i32})
                    n193 = call "Sequence.BuildPreviewWaveform.vi"("WaveformGraph in"=w523, "error in (no error)"=w520, "Rows"=w519, "UI.Sequence#ofColumns"=w524, "SequenceRef"=w515) -> ("error out"=w526:errorcluster, "Wavefrom"=w522:waveform(dbl)[])  [unwired: 5 in]
                  }
                }
                "Graph" <- w499
              }
              frame Default {
              }
            }
          }
          frame Error {
            n194 = call <vilib>:"Simple Error Handler.vi"("error in (no error)"=w531) -> ("error out"=w532:errorcluster)  [unwired: 4 in, 4 out]
            n195 = call <vilib>:"Clear Errors.vi"("error in (no error)"=w532) -> ("error out"=w530:errorcluster)  [unwired: 6 in]
          }
        }
      }
    }
    frame Error {
      n196 = disable-structure shown="Enabled" {
        frame Enabled {
          n197 = invoke class="VI" method="FP.Close"() -> ()  [unwired: 3 in, 3 out]
        }
        frame Disabled {
        }
      }
      n198 = One Button Dialog(message="NI VeriStand is not open. Please open NI VeriStand before running this utility.") -> ()  [unwired: 1 in, 1 out]
    }
  }
